vi "Bioinspired Stabilizing System Dynamic Modeling and Control of  a Gimbal System.vi"() -> ()   [LabVIEW 2021]
uses:
  <vilib>/MakerHub/LINX/Public/Sensors/Accelerometer/MPU60X0/DeviceAddresses.ctl
  <vilib>/MakerHub/LINX/Public/Sensors/Accelerometer/MPU60X0/GyroFullScaleRanges.ctl
  <vilib>/Simulation/Scripting/Companion Diagram/SimConfigNode/SimParams.ctl
  <vilib>/Simulation/Scripting/Companion Diagram/SimConfigNode/_simSolvers.ctl
  <vilib>/Simulation/Implementation/Shared/SIMSCR Execution Mode.ctl
  <vilib>/Simulation/Param Hierarchy/Typedefs/SIMPH Param Control Actions.ctl
  <vilib>/Simulation/Implementation/Shared/SIM limit type.ctl
  <vilib>/Simulation/Implementation/Shared/NILVSim_ParamChanged.vi
  <vilib>/Simulation/Implementation/Shared/NILVSIM_BeginStep.vi
  <vilib>/Simulation/SignalArithmetic/Implementation/NILVSim Gain.llb/SIM Gain (scalar).vi
  <vilib>/Simulation/ContinuousLinear/Implementation/NILVSim Derivative.llb/SIM derivative (scalar).vi
  <vilib>/Simulation/ContinuousLinear/Implementation/NILVSim Integrator new.llb/SIM Integrator distributor (scalar).vi
  <vilib>/Simulation/ContinuousLinear/Implementation/NILVSim Integrator new.llb/SIM Integrator collector (scalar).vi
  <vilib>/Simulation/Implementation/Shared/SIM Is Init or Final Stage.vi
  <vilib>/Simulation/Nonlinear/Implementation/NILVSim Saturation.llb/SIM Saturation (scalar).vi
  <vilib>/Simulation/Implementation/Shared/NILVSim_Manager.vi
  <vilib>/Utility/error.llb/Clear Errors.vi
  <vilib>/Simulation/Implementation/Shared/NILVSim_FinalizeModel.vi
  <vilib>/MakerHub/LINX/Public/Peripherals/Analog/Analog Read 1 Chan.vi
  <vilib>/MakerHub/LINX/Public/Peripherals/Analog/Analog Read N Chans.vi
  <vilib>/MakerHub/LINX/Private/Local IO/LinxAnalogRead.vi
  <vilib>/MakerHub/LINX/Public/Utilities/Check Channel.vi
  <vilib>/MakerHub/LINX/Public/Utilities/Open Serial.vi
  <vilib>/MakerHub/LINX/Public/Sensors/Motion/Servo/Servo Open One Channel.vi
  <vilib>/Simulation/Implementation/Shared/SIM Unbundle Sim Info.vi
  <vilib>/Simulation/Implementation/Shared/NILVSim_Initialize.vi
  <vilib>/Simulation/Utility/Implementation/NILVSim Get Time and IsAcceptedStep.vi
  <vilib>/Simulation/Implementation/Shared/SIMSH Read Queue.vi
  <vilib>/Simulation/Implementation/Shared/NILVSim_GetModelError.vi
  <vilib>/Simulation/Implementation/Shared/SIM Bundle Sim Info.vi
  <vilib>/MakerHub/LINX/Public/Sensors/Motion/Servo/Servo Set Pulse Width One Channel.vi
  <vilib>/MakerHub/LINX/Private/Utilties/Generate Error.vi
  <vilib>/MakerHub/LINX/Public/Sensors/Motion/Servo/Servo Close One Channel.vi
  <vilib>/Simulation/Scripting/Companion Diagram/SimConfigNode/SimDog.xnode
  <vilib>/Simulation/Implementation/XNodeFramework/SimXNode/SimX.xnode
  <vilib>/MakerHub/LINX/LMH-LINX.lvlib
  <vilib>/MakerHub/LINX/Public/Sensors/Accelerometer/MPU60X0/MPU60X0.lvlib
  <vilib>/MakerHub/LINX/Public/Sensors/Motion/Servo/Servo.lvlib
  <vilib>/ptbypt/NI_PtbyPt.lvlib
  <vilib>/Simulation/ContinuousLinear/Implementation/NILVSim Integrator new.llb/SIM Integrator (scalar).vi
  <vilib>/Simulation/Implementation/Shared/NI_SIM_Implementation.lvlib
panel:
  in  "Kd":dbl=1.58
  in  "Ki":dbl=0.013
  in  "Kp":dbl=1.5
  in  "Ki":dbl=0.014
  in  "Kd":dbl=0.214
  in  "Kp":dbl=1.58
  in  "ki 3":dbl=0.02
  in  "kd 3":dbl=0.2
  out "roll control":dbl=1607.490159902791
  in  "kp 3":dbl=2.3
  out "pitch control":dbl=1565.0465678888359
  out "yaw control":dbl=1587.1135373355996
  in  "initialize":bool
  in  "z-offset":i16=-100
  in  "y-offset":i16=130
  in  "x-offset":i16=325
  out "X Axis":i16=-1013
  out "yaw gyro":dbl=203.52648600508905 format="%0.2f"
  out "pitch gyro":dbl=152.8705699745547 format="%0.2f"
  out "roll gyro":dbl=174.21848346055975 format="%0.2f"
  out "pitch pos":dbl=134.764501953125
  out "roll pos":dbl=239.69970703125
  out "Yaw pos":dbl=194.95576171875
  out "Roll speed":dbl=1485.5973129770991
  out "Roll":dbl=-10.50381679389313
  out "Yaw":dbl=-234.9770992366412
  out "Pitch Speed":dbl=1514.9696396946565
  out "Pitch":dbl=10.473282442748092
  out "Yaw Speed":dbl=1851.777654961832
  in  "stop":bool
  out "Y-axis chart":dbl(graph)=10.473282442748092
  out "Z-axis Chart":dbl(graph)=-234.9770992366412
  out "X-axis Chart":dbl(graph)=-10.50381679389313
  in  "Gyro Full Scale Range":T1=enum."±500 °/s"
  in  "Baud Rate Override":u32=115200
  in  "Serial Port":refnum<visa-resource-name>="COM10"
  in  "I2C Slave Address":T2
  # "Pitch"
  # "Yaw"
  # "Roll"
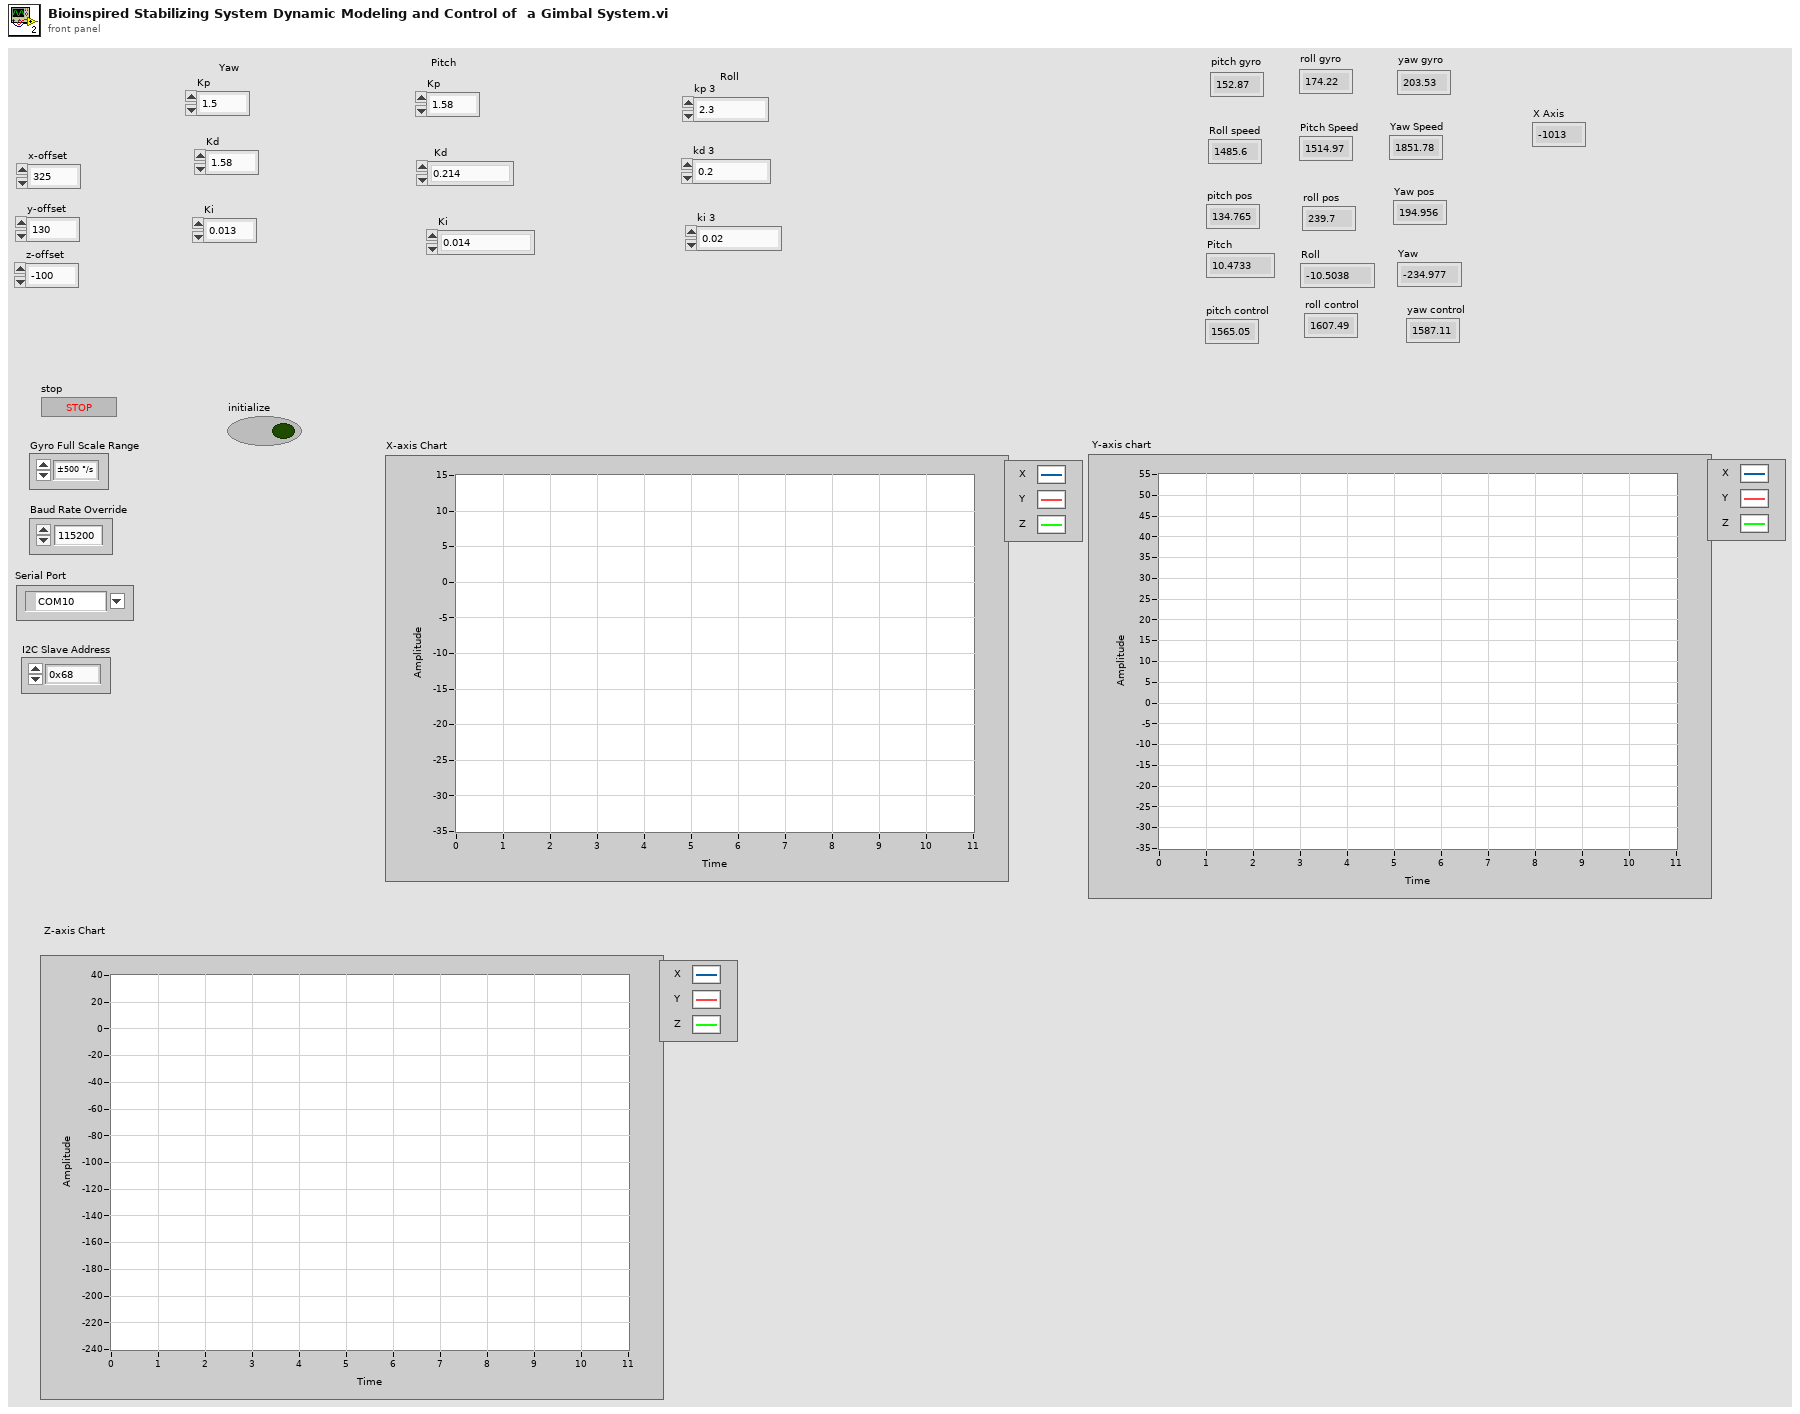
[diagram p1: front panel]
types:
  T1 = typedef "LMH-LINX.lvlib/MPU60X0.lvlib/GyroFullScaleRanges.ctl" = enum8{"±250 °/s", "±500 °/s", "±1000 °/s", "±2000 °/s"}
  T2 = typedef "LMH-LINX.lvlib/MPU60X0.lvlib/DeviceAddresses.ctl" = enum16{"0x68", "0x69"}
  T3 = typedef "LMH-LINX.lvlib/LINX Ref.ctl" = cluster{"IO":T4, "Interface":T5, "LINX Device Config":T6}
  T4 = typedef "LMH-LINX.lvlib/Platform.ctl" = enum16{"Remote", "Local"}
  T5 = typedef "LMH-LINX.lvlib/Interface.ctl" = enum16{"Serial", "TCP"}
  T6 = typedef "LMH-LINX.lvlib/Device.lvlib/LINX Device Config.ctl" = cluster{"Interface":T5, "COM Port":refnum<visa-resource-name>, "TCP Configuration":T7, "Device Family":u8, "Device ID":u8, "Device Name":string, "TCP Ref":refnum<k5>, "Channels":T8}
  T7 = typedef "LMH-LINX.lvlib/Device.lvlib/TCP Config.ctl" = cluster{"IP Address":string, "Port":u16}
  T8 = typedef "LMH-LINX.lvlib/Channels.ctl" = cluster{"DI":u8[], "DO":u8[], "AI":u8[], "AO":u8[], "PWM":u8[], "QE":u8[], "UART":u8[], "I2C 2":u8[], "SPI":u8[], "CAN":u8[], "Servo":u8[], "AI Ref (V)":dbl, "AI Resolution (Bits)":u8, "AO Ref (V)":dbl, "AO Resolution (Bits)":u8}
  T9 = typedef "SIMSCR Execution Mode.ctl" = enum16{"Simulate to Completion", "Single Time-Step Simulation (Fixed Step Only)"}
  T10 = typedef "SIMPH Param Control Actions.ctl" = enum16{"get params", "set params"}
  T11 = typedef "SIM limit type.ctl" = enum16{"upper", "lower", "both", "none"}
  T12 = typedef "SimParams.ctl" = cluster{"Initial Time (s)":dbl, "Final Time (s)":dbl, "Step Size (s)":dbl, "ODE Solver":T13, "Minimum Step Size (s)":dbl, "Maximum Step Size (s)":dbl, "Relative Tolerance":dbl, "Absolute Tolerance":dbl, "Software Timing":bool, "Initial Step Size (s)":dbl, "Automatic Fixed Step Size?":bool, "Automatic Discrete Step Size?":bool, "Discrete Step Size (s)":dbl, "Calculate using Time Step":bool, "Solver Wired?":bool, "Prev.Frm.Expected End":u64, "Prev.Frm.Actual End":u64, "Prev.Frm.Finished Late?":bool, "Prev.Iter.Expected End":u64, "Prev.Iter.Actual End":u64, "Prev.Iter.Finished Late?":bool, "Expected Iteration Start":u64, "Actual Iteration Start":u64, "Expected Frame Start":u64, "Actual Frame Start":u64, "Source Name":string, "Name":string, "Period":i64, "Deadline":i64, "Offset":i64, "Start":i64, "Priority":i32, "Timeout":i32, "Processor":i32, "Mode":enum32{"No Change", "Process missed periods, maintain original phase", "Discard missed periods, maintain original phase", "Process missed periods, ignore original phase", "Discard missed periods, ignore original phase"}, "Wakeup reason":enum32{"Normal", "Aborted", "Asynchronous wakeup", "Timing source error", "Timed loop error", "Timeout"}, "Error":errorcluster, "Source Type":string, "Secondary Source Type":string, "Global End Time":u64, "Global Start Time":u64, "Full Solver Reset":bool, "Execution Mode":T9, "Nan/Inf Check":bool, "Custom Solver Library":string, "Solver Is Variable":bool, "custom solver name":string, "Signal Collection Decimation":u32}
  T13 = typedef "_simSolvers.ctl" = enum16{"Runge-Kutta 1 (Euler)", "Runge-Kutta 2", "Runge-Kutta 3", "Runge-Kutta 4", "Runge-Kutta 23 (variable)", "Runge-Kutta 45 (variable)", "BDF (variable)", "Adams-Moulton (variable)", "Rosenbrock (variable)", "Discrete States Only", "SDIRK 4 (variable)", "Radau 5 (variable)", "Radau 9 (variable)", "Radau 13 (variable)", "Radau [Variable Order] (variable)", "Gear's Method (variable)", "Linearizer", "State Query", "Trim Eval", "Custom Solver"}
  T14 = cluster{"X Axis":i16, "Y Axis":i16, "Z Axis":i16}
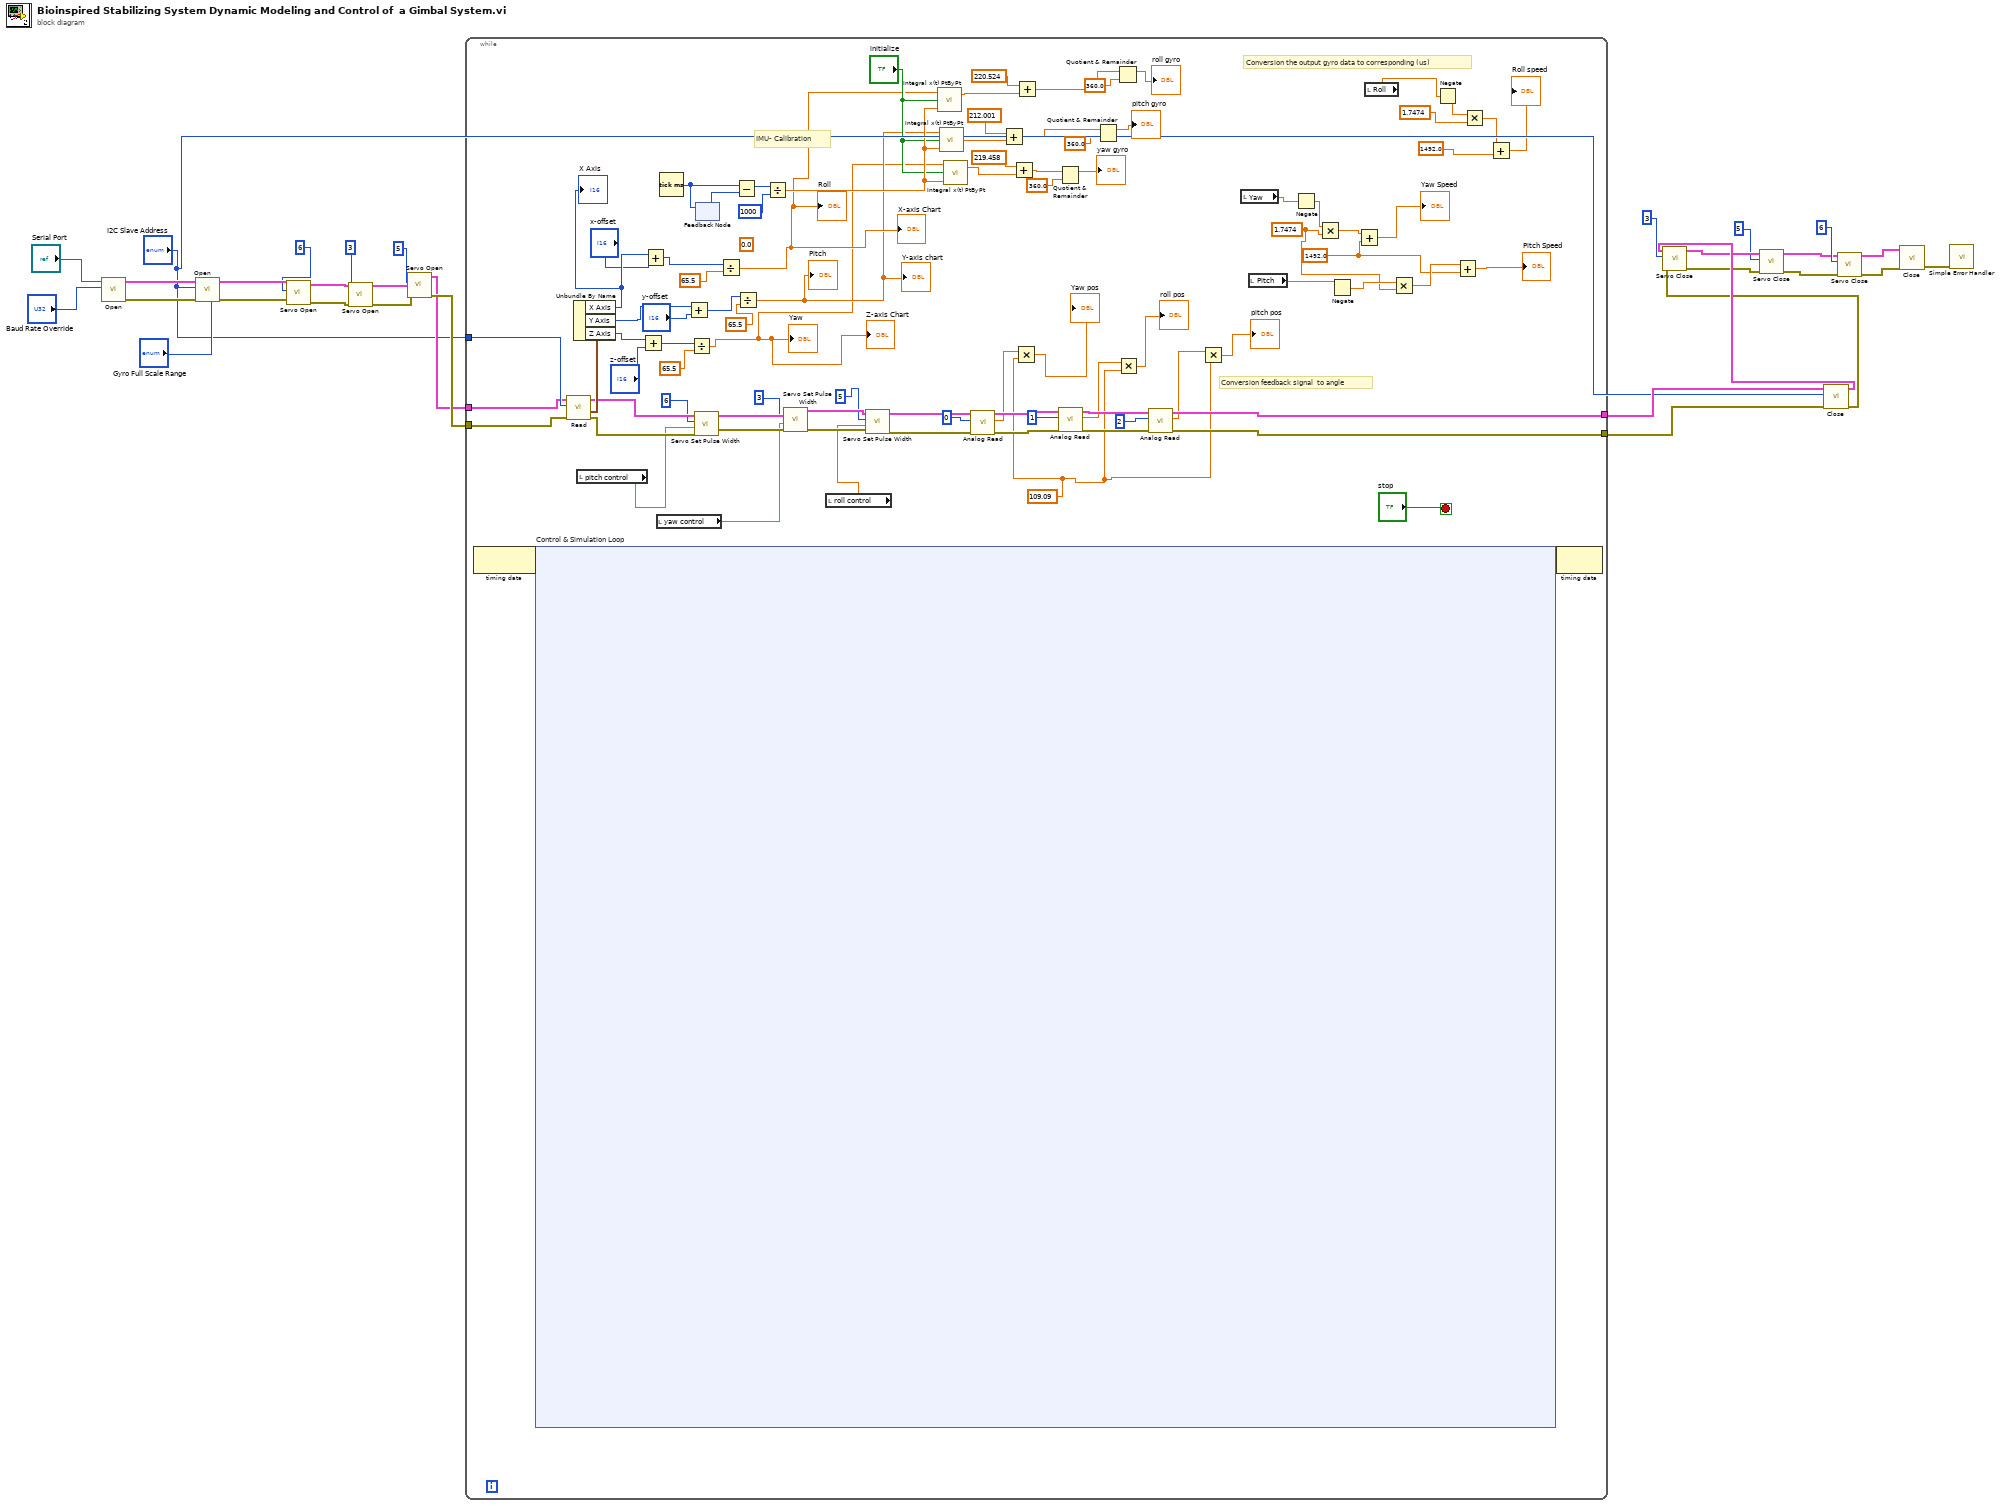
[diagram p0: block diagram]
diagram:
  n1 = call-poly <vilib>:"Open.vi"("Baud Rate Override"="Baud Rate Override", "Serial Port"="Serial Port") -> ("Error Out"=w26:errorcluster, "LINX Resource"=w27:T3)  [unwired: 7 in, 1 out]
  n2 = call <vilib>:"Open.vi"("Gyro Full Scale Range"="Gyro Full Scale Range", "Error In"=w26, "I2C Slave Address"="I2C Slave Address", "LINX Resource"=w27) -> ("Error Out"=w24:errorcluster, "LINX Resource"=w25:T3)  [unwired: 6 in]
  n3 = call-poly <vilib>:"Servo Open.vi"("Error In"=w24, "Servo Channel"=u8 6, "LINX Resource"=w25) -> ("Error Out"=w18:errorcluster, "LINX Resource"=w20:T3)  [unwired: 7 in]
  n4 = call-poly <vilib>:"Servo Open.vi"("Error In"=w18, "Servo Channel"=u8 3, "LINX Resource"=w20) -> ("Error Out"=w17:errorcluster, "LINX Resource"=w19:T3)  [unwired: 7 in]
  n5 = call-poly <vilib>:"Servo Open.vi"("Error In"=w17, "Servo Channel"=u8 5, "LINX Resource"=w19) -> ("Error Out"=w16:errorcluster, "LINX Resource"=w2:T3)  [unwired: 7 in]
  n6 = while {
    tunnel: "I2C Slave Address" -> [w120]
    tunnel: w2 -> [w100]
    tunnel: w16 -> [w99]
    tunnel: [w78] -> w4
    tunnel: [w77] -> w3
    stop <- "stop" stop-if-true
    w68 = 109.09
    w83 = 1.7474 ("x")
    w82 = 1492.0 ("y")
    (unwired) 0.0 ("y")
    # "IMU- Calibration"
    # "Conversion the output gyro data to corresponding (us)"
    # "Conversion feedback signal  to angle"
    n7 = node-c288() -> (w48:variant)  [unwired: 1 in]
    n8 = node-c254 "Control & Simulation Loop"(w48) -> (w47:variant)
    n9 = call <vilib>:"Read.vi"("Error In"=w99, "I2C Slave Address"=w120, "LINX Resource"=w100) -> ("Error Out"=w104:errorcluster, "Gyro  Data (dps)"=w118:T14, "LINX Resource"=w105:T3)  [unwired: 4 in, 2 out]
    n10 = Unbundle By Name(w118) -> ("X Axis"=w117:i16, "Y Axis"=w103:i16, "Z Axis"=w114:i16)
    "X Axis" <- w117
    n11 = local read "pitch control"() -> (w42:dbl)
    n12 = Add(x=w114, y="z-offset") -> (x+y=w108:i16)
    n13 = Add(x=w117, y="x-offset") -> (x+y=w112:i16)
    n14 = local read "yaw control"() -> (w46:dbl)
    n15 = Tick Count (ms)() -> (millisecond timer value=w59:u32)
    n16 = Add(x=w103, y="y-offset") -> (x+y=w110:i16)
    n17 = Divide(x=w108, y=65.5) -> (x/y=w35:dbl)
    "Z-axis Chart" <- w35
    "Yaw" <- w35
    n18 = call-poly <vilib>:"Servo Set Pulse Width.vi"("Error In"=w104, "Pulse Width (uS)"=w42, "Servo Channel"=u8 6, "LINX Resource"=w105) -> ("Error Out"=w94:errorcluster, "LINX Resource"=w97:T3)  [unwired: 6 in]
    n19 = feedback-in #1(w59) -> ()
    n20 = feedback #1() -> (w60:u32)  [unwired: 1 in]
    n21 = Divide(x=w112, y=65.5) -> (x/y=w43:dbl)
    "X-axis Chart" <- w43
    "Roll" <- w43
    n22 = Subtract(x=w59, y=w60) -> (x-y=w58:u32)
    n23 = Divide(x=w110, y=65.5) -> (x/y=w36:dbl)
    "Y-axis chart" <- w36
    "Pitch" <- w36
    n24 = Divide(x=w58, y=u32 1000) -> (x/y=w56:dbl)
    n25 = call-poly <vilib>:"Servo Set Pulse Width.vi"("Error In"=w94, "Pulse Width (uS)"=w46, "Servo Channel"=u8 3, "LINX Resource"=w97) -> ("Error Out"=w95:errorcluster, "LINX Resource"=w96:T3)  [unwired: 6 in]
    n26 = local read "roll control"() -> (w41:dbl)
    n27 = call-poly <vilib>:"Servo Set Pulse Width.vi"("Error In"=w95, "Pulse Width (uS)"=w41, "Servo Channel"=u8 5, "LINX Resource"=w96) -> ("Error Out"=w74:errorcluster, "LINX Resource"=w81:T3)  [unwired: 6 in]
    n28 = call <vilib>:"Integral x(t) PtByPt.vi"("initialize"="initialize", "dt"=w56, "x"=w43) -> ("integral x(t)"=w54:dbl)  [unwired: 1 in, 1 out]
    n29 = call <vilib>:"Integral x(t) PtByPt.vi"("initialize"="initialize", "dt"=w56, "x"=w36) -> ("integral x(t)"=w52:dbl)  [unwired: 1 in, 1 out]
    n30 = call <vilib>:"Integral x(t) PtByPt.vi"("initialize"="initialize", "dt"=w56, "x"=w35) -> ("integral x(t)"=w50:dbl)  [unwired: 1 in, 1 out]
    n31 = call-poly <vilib>:"Analog Read.vi"("Error In"=w74, "Analog Channel"=u8 0, "LINX Resource"=w81) -> ("Error Out"=w75:errorcluster, "Voltage"=w70:dbl, "LINX Resource"=w80:T3)  [unwired: 5 in, 1 out]
    n32 = Add(x=212.001, y=w52) -> (x+y=w39:dbl)
    n33 = Add(x=219.458, y=w50) -> (x+y=w45:dbl)
    n34 = Multiply(x=w70, y=w68) -> (x*y=→"Yaw pos":dbl)
    n35 = Add(x=220.524, y=w54) -> (x+y=w37:dbl)
    n36 = Quotient & Remainder(x=w45, y=360.0) -> (x-y*floor(x/y)=→"yaw gyro":dbl)  [unwired: 1 out]
    n37 = call-poly <vilib>:"Analog Read.vi"("Error In"=w75, "Analog Channel"=u8 1, "LINX Resource"=w80) -> ("Error Out"=w76:errorcluster, "Voltage"=w69:dbl, "LINX Resource"=w79:T3)  [unwired: 5 in, 1 out]
    n38 = Quotient & Remainder(x=w39, y=360.0) -> (x-y*floor(x/y)=→"pitch gyro":dbl)  [unwired: 1 out]
    n39 = Quotient & Remainder(x=w37, y=360.0) -> (x-y*floor(x/y)=→"roll gyro":dbl)  [unwired: 1 out]
    n40 = Multiply(x=w69, y=w68) -> (x*y=→"roll pos":dbl)
    n41 = call-poly <vilib>:"Analog Read.vi"("Error In"=w76, "Analog Channel"=u8 2, "LINX Resource"=w79) -> ("Error Out"=w77:errorcluster, "Voltage"=w67:dbl, "LINX Resource"=w78:T3)  [unwired: 5 in, 1 out]
    n42 = Multiply(x=w67, y=w68) -> (x*y=→"pitch pos":dbl)
    n43 = local read "Yaw"() -> (w91:dbl)
    n44 = local read "Pitch"() -> (w87:dbl)
    n45 = Negate(x=w91) -> (-x=w90:dbl)
    n46 = Multiply(x=w90, y=w83) -> (x*y=w106:dbl)
    n47 = Negate(x=w87) -> (-x=w86:dbl)
    n48 = Add(x=w106, y=w82) -> (x+y=→"Yaw Speed":dbl)
    n49 = local read "Roll"() -> (w89:dbl)
    n50 = Multiply(x=w86, y=w83) -> (x*y=w102:dbl)
    n51 = Negate(x=w89) -> (-x=w88:dbl)
    n52 = Add(x=w102, y=w82) -> (x+y=→"Pitch Speed":dbl)
    n53 = Multiply(x=w88, y=1.7474 ("x")) -> (x*y=w101:dbl)
    n54 = Add(x=w101, y=1492.0) -> (x+y=→"Roll speed":dbl)
    n55 = node-c288(w47) -> ()  [unwired: 1 out]
  }
  n56 = call <vilib>:"Close.vi"("Error In"=w3, "I2C Slave Address (0)"="I2C Slave Address", "LINX Resource"=w4) -> ("Error Out"=w9:errorcluster, "LINX Resource"=w14:T3)  [unwired: 7 in]
  n57 = call-poly <vilib>:"Servo Close.vi"("Error In"=w9, "Servo Channel"=u8 3, "LINX Resource"=w14) -> ("Error Out"=w10:errorcluster, "LINX Resource"=w13:T3)  [unwired: 7 in]
  n58 = call-poly <vilib>:"Servo Close.vi"("Error In"=w10, "Servo Channel"=u8 5, "LINX Resource"=w13) -> ("Error Out"=w11:errorcluster, "LINX Resource"=w12:T3)  [unwired: 7 in]
  n59 = call-poly <vilib>:"Servo Close.vi"("Error In"=w11, "Servo Channel"=u8 6, "LINX Resource"=w12) -> ("Error Out"=w22:errorcluster, "LINX Resource"=w21:T3)  [unwired: 7 in]
  n60 = call <vilib>:"Close.vi"("Error In"=w22, "LINX Resource"=w21) -> ("Error Out"=w31:errorcluster)  [unwired: 9 in]
  n61 = call <vilib>:"Simple Error Handler.vi"("error in (no error)"=w31) -> ()  [unwired: 4 in, 5 out]
